vi "Matrix left divisionMM_general_direct.vi"(2 "A":dbl[][](array[numeric]), 4 "B":dbl[][](array[numeric])) -> (0 "error":i32, 1 "B\\A":dbl[][](array[numeric]))   [LabVIEW 2014, in "NI_Gmath.lvlib"]
doc: "Left division operator. B\\A solves the equation B*X=A. When used with two polynomials, \\ is overloaded to produce a transfer function whose numerator is the right-hand operand. When used with two dynamic systems, a new system is created whose state matrix is the appended states of the two systems and whose output matrix is that of the \"numerator\" system. (For systems in transfer- function format, the new system is obtained by multiplying the \"numerator\" system by the reciprocal of the \"denominator\" system.) For matrix division, there are no specific conditions on the dimensions of A and B but the condition of B affects the accuracy of the matrix quotient obtained. An error message appears if B is singular. If B is square and nonsingular, B\\A returns a matrix X with the same dimensions as A. An LU (Gaussian) decomposition, rather than a direct inverse, is used. If the condition estimate of B is less than the machine epsilon, a warning message appears. If B is non-square, X is the least-squares solution to B*X=A and has row dimension equal to the number of columns of B and column dimension equal to the number of columns of A. This operation uses a QR decomposition to implicitly compute the rank of B; the solution X will have no more nonzero components in each column than this rank value."
uses:
  NI_Gmath.lvlib
  Real PseudoInverse Matrix.vi
  Real A x B.vi
  NI_AALBase.lvlib
  NI_AALPro.lvlib
  lvanlys.dll
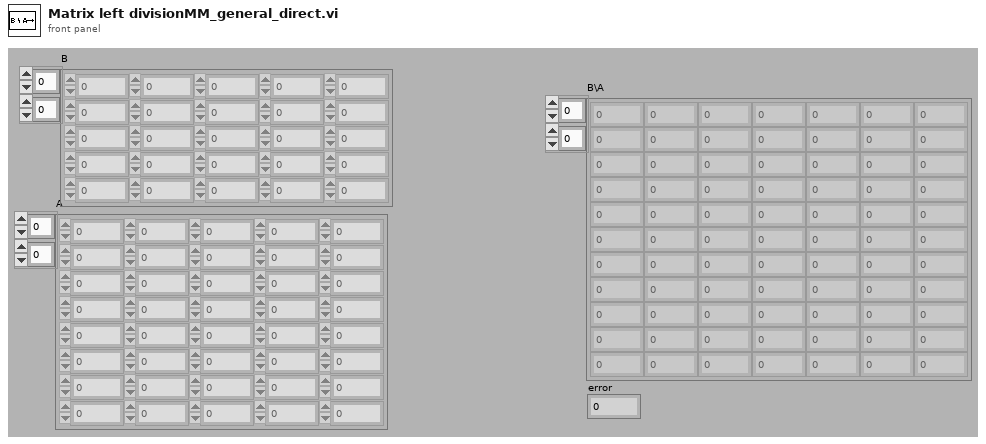
[diagram p1: front panel]
types:
  T1 = typedef "NI_Matrix.lvlib/RealMatrix.ctl" = dbl[][]
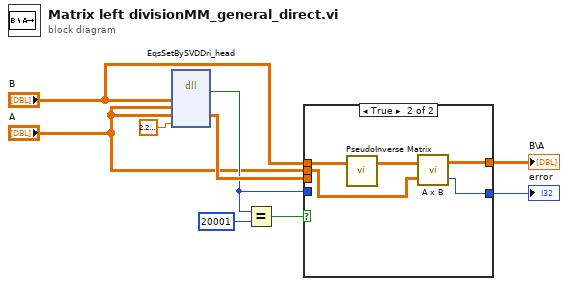
[diagram p0: block diagram]
diagram:
  n1 = dll-call lib="C:/Program Files (x86)/National Instruments/LabVIEW 2014/resource/lvanlys.*" fn="EqsSetBySVDDri_head"("aH"="B", "bH"="A", "xH"="A", "relativeTol"=2.220446049250313e-16) -> ("return type"=w4:i32, "xH"=w5:dbl[][])  [unwired: 6 in, 2 out]
  n2 = Equal?(x=w4, y=20001) -> (x = y?=w6:bool)
  n3 = case shown="True" w6 {
    tunnel: "B" -> [_ w16]
    tunnel: [w10 w13] -> w8
    tunnel: [w11 w14] -> w9
    tunnel: w4 -> [w11 _]
    tunnel: w5 -> [w10 _]
    tunnel: "A" -> [_ w12]
    frame False {
    }
    frame True {
      n4 = call-poly "PseudoInverse Matrix.vi"("Input Matrix"=w16) -> ("PseudoInverse Matrix"=w15:T1)  [unwired: 1 in, 1 out]
      n5 = call-poly "A x B.vi"("B"=w12, "A"=w15) -> ("error"=w14:i32, "A x B"=w13:T1)
    }
  }
  "B\\A" <- w8
  "error" <- w9
